vi "setTheme.Colors.vi"(10 "Colors":T1, 11 "Filled Text Fields Actor in":refnum<class "Filled Text Fields Actor.lvclass">) -> (3 "Filled Text Fields Actor out":refnum<class "Filled Text Fields Actor.lvclass">)   [LabVIEW 2017, in "Filled Text Fields.lvlib" / "Filled Text Fields Actor.lvclass"]
uses:
  Filled Text Fields Actor.lvclass
  Theme/Theme.Colors/Colors.ctl
  Filled Text Fields Actor.lvclass/Filled Text Fields Actor.ctl
  Theme/Theme/setColors.vi
  Theme/Theme/Theme.lvclass
  Theme/Theme.Colors/Theme.Colors.lvclass
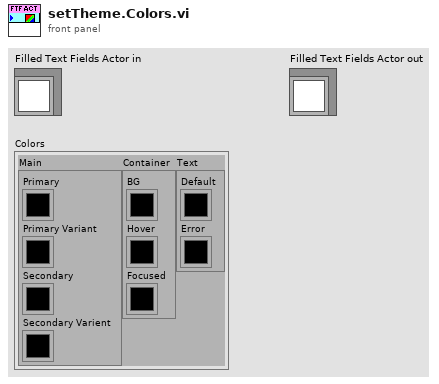
[diagram p1: front panel]
types:
  T1 = typedef "Theme.lvlib/Theme.Colors.lvclass/Colors.ctl" = cluster{"Main":cluster{"Primary":u32, "Primary Variant":u32, "Secondary":u32, "Secondary Varient":u32}, "Container":cluster{"BG":u32, "Hover":u32, "Focused":u32}, "Text":cluster{"Default":u32, "Error":u32}}
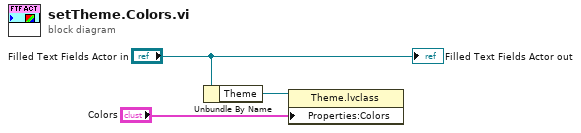
[diagram p0: block diagram]
diagram:
  n1 = Unbundle By Name("Filled Text Fields Actor in") -> ("Theme"=w2:refnum<class "Theme.lvclass">)
  n2 = property class="Theme.lvclass"(reference=w2, "Properties:Colors"="Colors") -> ()  [unwired: 1 in, 2 out]
  "Filled Text Fields Actor out" <- "Filled Text Fields Actor in"
